vi "Get Formatter.vi"(11 "Input String":string) -> (1 "Post Formatter":string, 2 "Formatter":string, 3 "Before Formatter":string)   [LabVIEW 2020, in "Composed Log.lvlib" / "LoggerReference.lvclass"]
uses:
  <vilib>/gpm_packages/@cs/event-logger/Source/Composed Log/LoggerReference/LoggerReference.lvclass
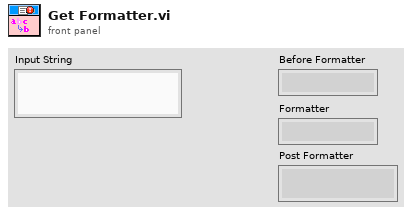
[diagram p1: front panel]
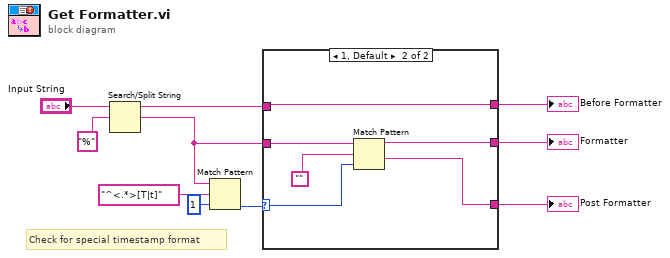
[diagram p0: block diagram]
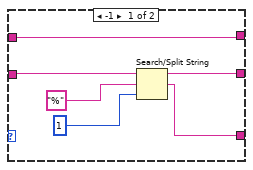
[diagram p2: hidden frame]
diagram:
  # "Check for special timestamp format"
  n1 = Search/Split String(string="Input String", search string/char (-)="%" ("regular expression")) -> (substring before match=w6:string, match + rest of string=w3:string)  [unwired: 1 in, 1 out]
  n2 = Match Pattern(string=w3, regular expression="^<.*>[T|t]", offset (0)=1) -> (offset past match=w2:i32)  [unwired: 3 out]
  n3 = case shown="1, Default" w2 {
    selector: w2 -> [_ w19]
    tunnel: [w11 w18] -> w10
    tunnel: [w12 w17] -> w9
    tunnel: w3 -> [w15 w21]
    tunnel: w6 -> [w16 w22]
    tunnel: [w16 w22] -> w5
    frame -1 {
      n4 = Search/Split String(string=w15, search string/char (-)="%", offset (0)=1) -> (substring before match=w11:string, match + rest of string=w12:string)  [unwired: 1 out]
    }
    frame 1, Default {
      n5 = Match Pattern(string=w21, regular expression="", offset (0)=w19) -> (before substring=w18:string, after substring=w17:string)  [unwired: 2 out]
    }
  }
  "Before Formatter" <- w5
  "Post Formatter" <- w9
  "Formatter" <- w10
